vi "Put Get over Mdsip Connection.vi"() -> ()   [LabVIEW 2015]
uses:
  Library/MDSplus.lvlib
panel:
  in  "Path":string
  in  "Data In":sgl
  in  "Shot":i32
  in  "Tree":string
  in  "Expression":string
  out "Data Out":sgl
  in  "IP:port":string
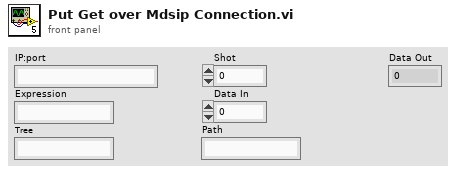
[diagram p1: front panel]
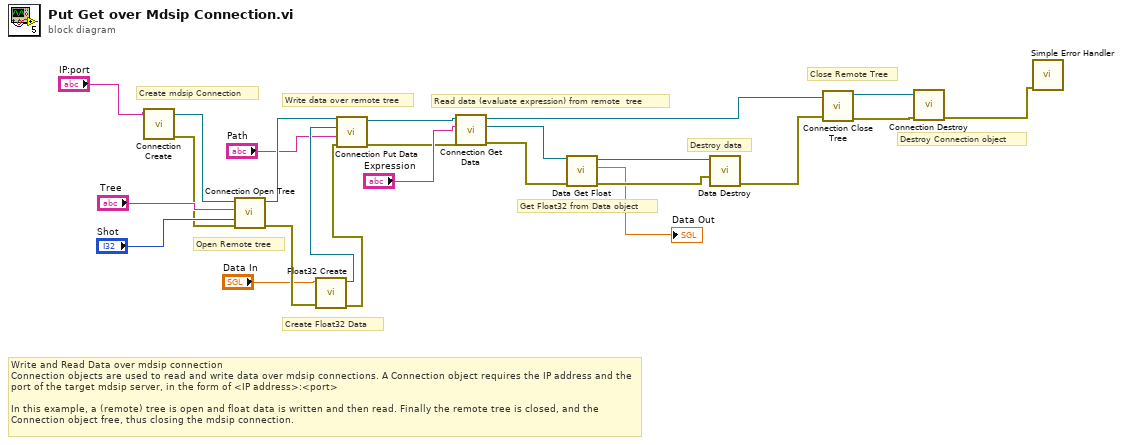
[diagram p0: block diagram]
diagram:
  # "Destroy Connection object"
  # "Close Remote Tree"
  # "Destroy data"
  # "Get Float32 from Data object"
  # "Read data (evaluate expression) from remote  tree"
  # "Write data over remote tree"
  # "Create Float32 Data"
  # "Open Remote tree"
  # "Create mdsip Connection"
  # "Write and Read Data over mdsip connection\nConnection objects are used to read and write data over mdsip connections. A Connection object requires the IP address and the port of the target mdsip server, in the form of <IP address>:<port>\n\nIn this example, a (remote) tree is open and float data is written and then read. Finally the remote tree is closed, and the Connection object free, thus closing the mdsip connection."
  n1 = call "Connection Create.vi"("Ip : port"="IP:port") -> ("error out"=w1:errorcluster, "Connection DVR out"=w22:refnum<data-value>)  [unwired: 9 in]
  n2 = call "Connection Open Tree.vi"("error in (no error)"=w1, "Shot"="Shot", "Tree"="Tree", "Connection DVR in"=w22) -> ("error out"=w19:errorcluster, "Connection DVR out"=w17:refnum<data-value>)  [unwired: 6 in]
  n3 = call "Float32 Create.vi"("error in (no error)"=w19, "SGL in"="Data In") -> ("error out"=w16:errorcluster, "Float32 DVR out"=w15:refnum<data-value>)  [unwired: 8 in]
  n4 = call "Connection Put Data.vi"("error in (no error)"=w16, "Path in"="Path", "Data"=w15, "Connection DVR in"=w17) -> ("error out"=w12:errorcluster, "Connection DVR out"=w13:refnum<data-value>)  [unwired: 6 in]
  n5 = call "Connection Get Data.vi"("error in (no error)"=w12, "Expression in"="Expression", "Connection DVR in"=w13) -> ("error out"=w9:errorcluster, "Data DVR out"=w11:refnum<data-value>, "Connection DVR out"=w4:refnum<data-value>)  [unwired: 6 in]
  n6 = call "Data Get Float.vi"("error in (no error)"=w9, "Data DVR in"=w11) -> ("error out"=w8:errorcluster, "SGL out"=→"Data Out":sgl, "Data DVR out"=w10:refnum<data-value>)  [unwired: 7 in]
  n7 = call "Data Destroy.vi"("error in (no error)"=w8, "Data DVR in"=w10) -> ("error out"=w3:errorcluster)  [unwired: 9 in]
  n8 = call "Connection Close Tree.vi"("error in (no error)"=w3, "Connection DVR in"=w4) -> ("error out"=w2:errorcluster, "Connection DVR out"=w5:refnum<data-value>)  [unwired: 8 in]
  n9 = call "Connection Destroy.vi"("error in (no error)"=w2, "Connection DVR in"=w5) -> ("error out"=w6:errorcluster)  [unwired: 9 in]
  n10 = call <vilib>:"Simple Error Handler.vi"("error in (no error)"=w6) -> ()  [unwired: 4 in, 5 out]
